vi "sub_trigger-checkforstart2.vi"(7 "check":enum16{"check", "clear"}(ring), 11 "Waveform":waveform(dbl)) -> (0 "result array":bool[](array[boolean]), 1 "stop trg":bool, 2 "start trg":bool, 3 "trigger":bool)   [LabVIEW 2013]
uses:
  <vilib>/Analysis/baseanly.llb/Mean (DBL).vi
  <vilib>/measure/madcrms.llb/Basic Averaged DC-RMS for 1 Chan.vi
  <vilib>/measure/mamon.llb/Trigger Detection for 1 Channel.vi
  <vilib>/measure/NI_MAPro.lvlib
  <vilib>/Analysis/NI_AALBase.lvlib
panel:
  in  "trg flag":cluster{"start":bool, "stop":bool, "high":bool}
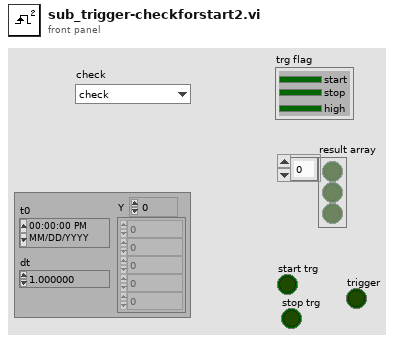
[diagram p1: front panel]
types:
  T1 = typedef "config_ctl.ctl" = cluster{"Trigger minlevel":dbl, "Lower Cut-Off":dbl, "Vacuum Trigger level":dbl, "state settings":cluster{"method":enum32{"histogram", "peak", "auto select"}, "histogram size":i32, "histogram method":enum16{"mode"}, "reserved":dbl}, "SPA-300 Setting":cluster{"Bonding force (g)":dbl, "Bonding time (ms)":dbl, "Pickup force (g)":dbl, "Pickup time (ms)":dbl, "Speed":enum16{"Slow", "Fast"}}}
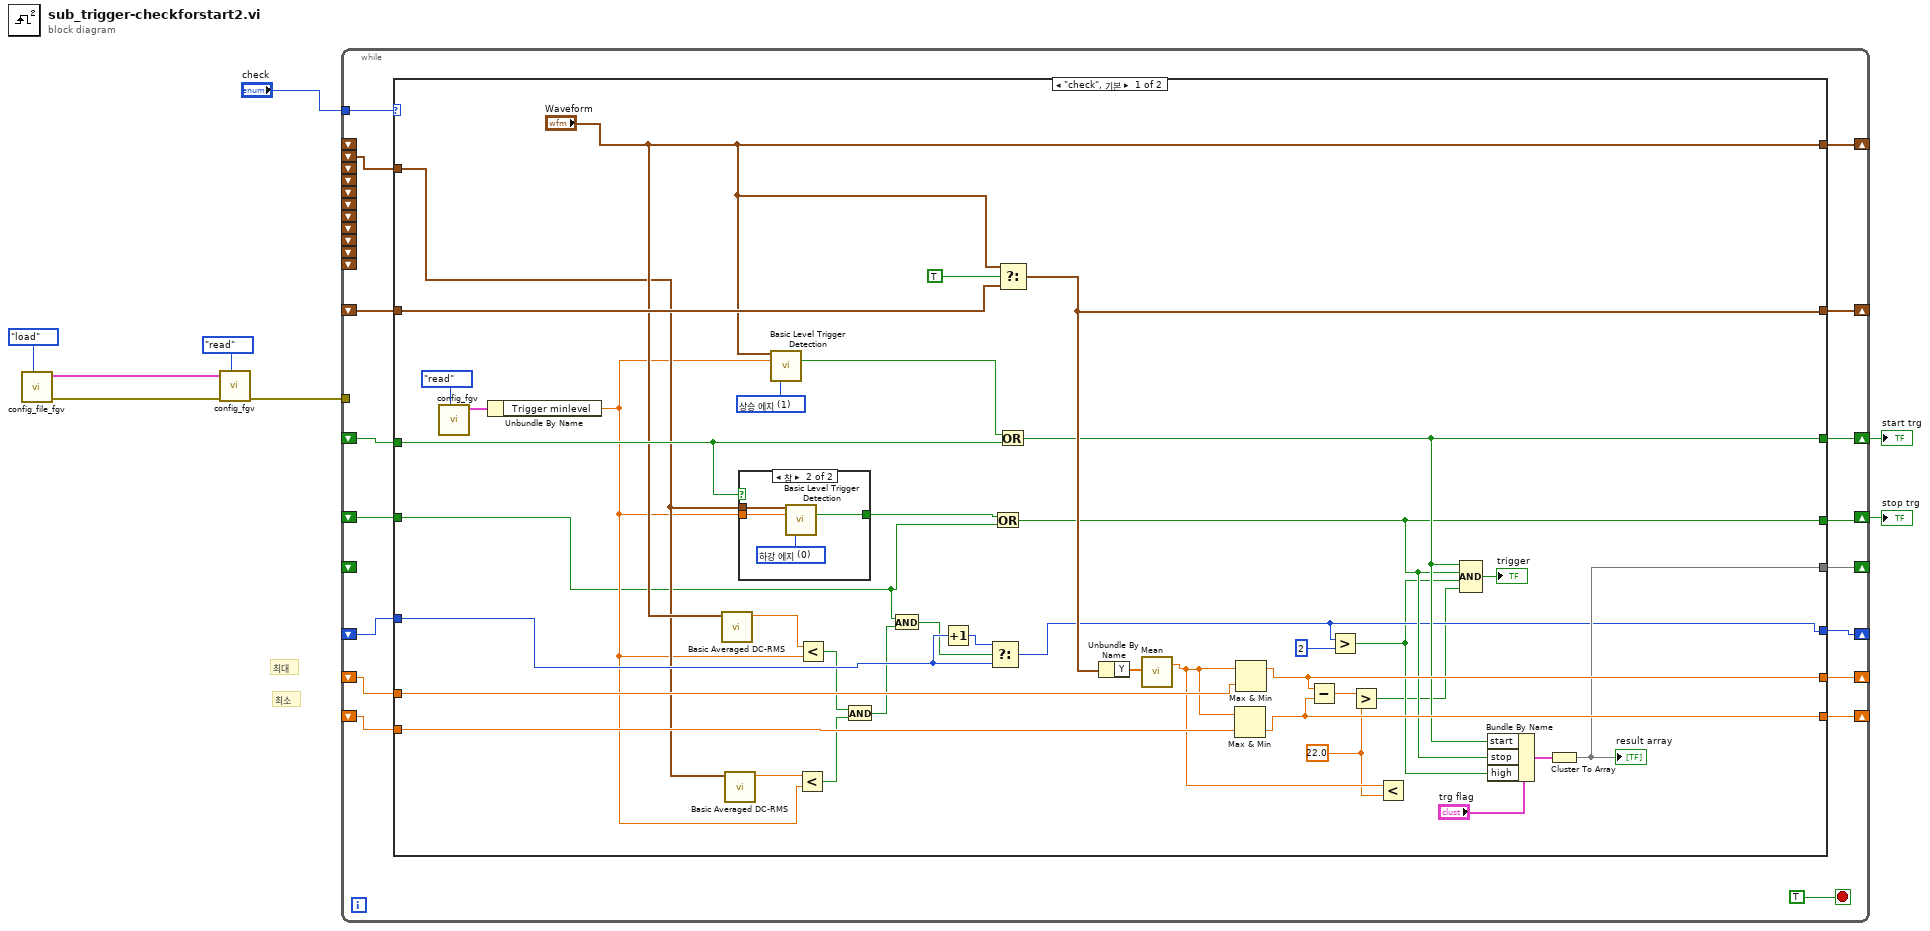
[diagram p0: block diagram]
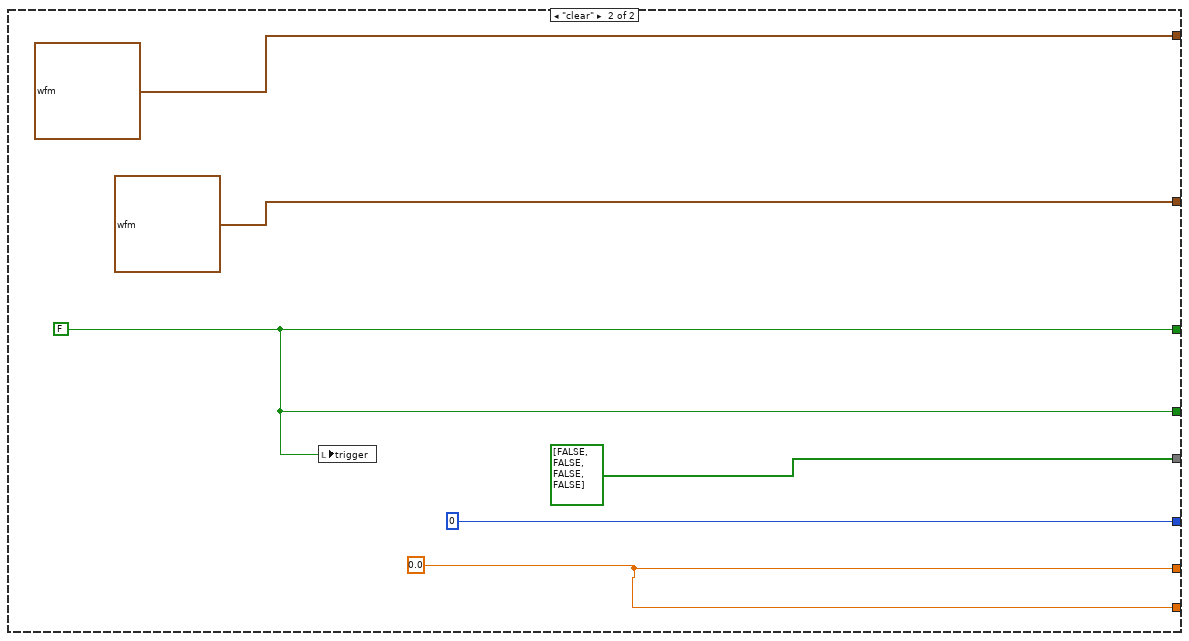
[diagram p3: hidden frame]
diagram:
  # "최소"
  # "최대"
  n1 = call "config_file_fgv.vi"("cmd"=enum16{"save", "load"}."load") -> ("error out"=w1:errorcluster, "var"=w2:T1)  [unwired: 8 in, 1 out]
  n2 = call "config_fgv.vi"("cmd"=enum16{"write", "read", "ini"}."read", "error in (no error)"=w1, "Config in"=w2) -> ("error out"=w4:errorcluster)  [unwired: 7 in, 1 out]
  n3 = while {
    shift-right: [w23] -> w7
    shift-left: _ -> [w22]
    tunnel: "check" -> [w24]
    shift-right: [w21] -> _
    shift-left: _ -> [_]
    shift-left: _ -> [w9]
    shift-left: _ -> [_]
    shift-right: [w20] -> w6
    shift-left: _ -> [w19]
    shift-right: [w18] -> _
    shift-left: _ -> [w17]
    shift-right: [w14] -> _
    shift-left: _ -> [w16]
    shift-right: [w13] -> _
    shift-left: _ -> [w15]
    shift-right: [w12] -> _
    shift-left: _ -> [_]
    shift-left: _ -> [_]
    shift-left: _ -> [_]
    shift-left: _ -> [_]
    shift-left: _ -> [_]
    shift-left: _ -> [_]
    shift-left: _ -> [_]
    shift-left: _ -> [_]
    shift-left: _ -> [_]
    shift-right: [w11] -> _
    shift-left: _ -> [w10]
    tunnel: w4 -> [_]
    stop <- TRUE stop-if-true
    n4 = case shown="\"check\", 기본" w24 {
      tunnel: [w47 w73] -> w23
      tunnel: w22 -> [w60 _]
      tunnel: ["Waveform" waveform(dbl) {"t0"=timestamp(0 s since 1904-01-01), "dt"=0.00062, "Y"=[]} ("Waveform")] -> w21
      tunnel: w9 -> [w33 _]
      tunnel: [w46 w73] -> w20
      tunnel: w19 -> [w28 _]
      tunnel: [w59 waveform(dbl) {"t0"=timestamp(0 s since 1904-01-01), "dt"=0.00062, "Y"=[]} ("Waveform")] -> w18
      tunnel: w17 -> [w61 _]
      tunnel: w16 -> [w57 _]
      tunnel: w15 -> [w56 _]
      tunnel: [w55 w72] -> w14
      tunnel: [w54 w72] -> w13
      tunnel: [w44 bool[] [FALSE, FALSE, FALSE, FALSE]] -> w12
      tunnel: [w38 0] -> w11
      tunnel: w10 -> [w40 _]
      frame "check", Default {
        w50 = 22.0 ("y")
        w64 = u16 1 items=["하강 에지", "상승 에지"] ("trigger slope")
        n5 = call "config_fgv.vi"("cmd"=enum16{"write", "read", "ini"}."read") -> ("Config out"=w43:T1)  [unwired: 9 in, 1 out]
        n6 = Unbundle By Name(w43) -> ("Trigger minlevel"=w31:dbl)
        n7 = call-poly <vilib>:"Basic Averaged DC-RMS.vi"("signal in"="Waveform") -> ("DC value"=w41:dbl)  [unwired: 7 in, 3 out]
        n8 = call-poly <vilib>:"Basic Averaged DC-RMS.vi"("signal in"=w33) -> ("DC value"=w32:dbl)  [unwired: 7 in, 3 out]
        n9 = case shown="참" w60 {
          tunnel: [_ w67] -> w62
          tunnel: w33 -> [_ w66]
          tunnel: w31 -> [_ w65]
          frame False {
          }
          frame True {
            w68 = u16 0 items=["하강 에지", "상승 에지"] ("trigger slope")
            n10 = call-poly <vilib>:"Basic Level Trigger Detection.vi"("signal in"=w66, "level"=w65, "trigger slope"=w68) -> ("trigger detected?"=w67:bool)  [unwired: 10 in, 2 out]
          }
        }
        n11 = call-poly <vilib>:"Basic Level Trigger Detection.vi"("signal in"="Waveform", "level"=w31, "trigger slope"=w64) -> ("trigger detected?"=w63:bool)  [unwired: 10 in, 2 out]
        n12 = Less?(x=w32, y=w31) -> (x < y?=w30:bool)
        n13 = Less?(x=w41, y=w31) -> (x < y?=w29:bool)
        n14 = And(x=w29, y=w30) -> (x .and. y?=w27:bool)
        n15 = And(x=w28, y=w27) -> (x .and. y?=w26:bool)
        n16 = Increment(x=w40) -> (x+1=w39:i32)
        n17 = Select(t=w39, s=w26, f=w40) -> (s? t:f=w38:i32)
        n18 = Or(x=w62, y=w28) -> (x .or. y?=w46:bool)
        n19 = Select(t="Waveform", s=TRUE, f=w61) -> (s? t:f=w59:waveform(dbl))
        n20 = Or(x=w63, y=w60) -> (x .or. y?=w47:bool)
        n21 = Unbundle By Name(w59) -> ("Y"=w58:dbl[])
        n22 = call-poly <vilib>:"Mean.vi"("X"=w58) -> ("mean"=w51:dbl)  [unwired: 1 out]
        n23 = Max & Min(x=w51, y=w56) -> (min(x,y)=w54:dbl)  [unwired: 1 out]
        n24 = Max & Min(x=w51, y=w57) -> (max(x,y)=w55:dbl)  [unwired: 1 out]
        n25 = Subtract(x=w55, y=w54) -> (x-y=w53:dbl)
        n26 = Greater?(x=w38, y=2) -> (0:w36:bool)
        n27 = Greater?(x=w53, y=w50) -> (0:w35:bool)
        n28 = Less?(x=w51, y=w50) -> ()  [unwired: 1 out]
        n29 = Compound Arithmetic op=AND(w47, w46, w36, w35) -> (→"trigger":bool)
        n30 = Bundle By Name(cluster="trg flag", "start"=w47, "stop"=w46, "high"=w36) -> (w45:cluster{"start":bool, "stop":bool, "high":bool})
        n31 = Cluster To Array(cluster=w45) -> (array=w44:bool[])
        "result array" <- w44
      }
      frame "clear" {
        w72 = 0.0
        w73 = FALSE
        n32 = local write "trigger"(w73) -> ()
      }
    }
  }
  "start trg" <- w7
  "stop trg" <- w6
